vi "Write FPath+FExt.vi"(8 "error in (no error)":errorcluster, 9 "File Ext":string, 10 "File Path":path, 11 "Log in":refnum<class "Log.lvclass">) -> (0 "error out":errorcluster, 3 "Log out":refnum<class "Log.lvclass">)   [LabVIEW 2017, in "Report_lib.lvlib" / "Log.lvclass"]
uses:
  Log.lvclass
  Log.lvclass/Log.ctl
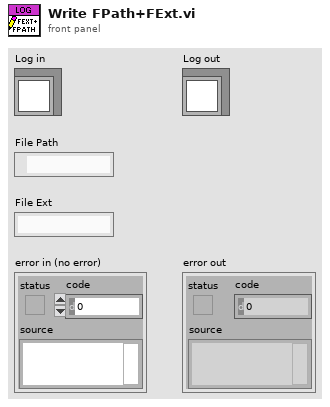
[diagram p1: front panel]
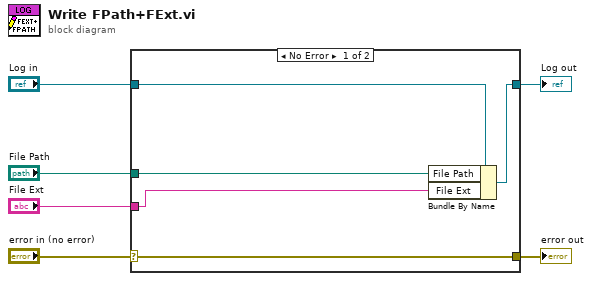
[diagram p0: block diagram]
diagram:
  n1 = case shown="No Error" "error in (no error)" {
    selector: "error in (no error)" -> [w11 w12]
    tunnel: [w11 w12] -> w5
    tunnel: [w9 w13] -> w3
    tunnel: "Log in" -> [w10 w13]
    tunnel: "File Path" -> [w8 _]
    tunnel: "File Ext" -> [w7 _]
    frame No Error {
      n2 = Bundle By Name(cluster=w10, "File Path"=w8, "File Ext"=w7) -> (w9:refnum<class "Log.lvclass">)
    }
    frame Error {
    }
  }
  "error out" <- w5
  "Log out" <- w3
